vi "Memory.Pointer.Write Bytes.Safe.vi"(8 "error in (no error)":errorcluster, 9 "offset (0)":u64 format="%d bytes", 10 "buffer":u8[](array[numeric]) format="%02x", 11 "Pointer in":refnum<class "Memory.Pointer.Void.lvclass">) -> (0 "error out":errorcluster, 1 "offset dup":u64 format="%d bytes", 2 "buffer dup":u8[](array[numeric]) format="%02x", 3 "Pointer out":refnum<class "Memory.Pointer.Void.lvclass">)   [LabVIEW 2016, in "Memory Manager.lvlib" / "Memory.Pointer.Void.lvclass"]
uses:
  Memory.Pointer.Void.lvclass
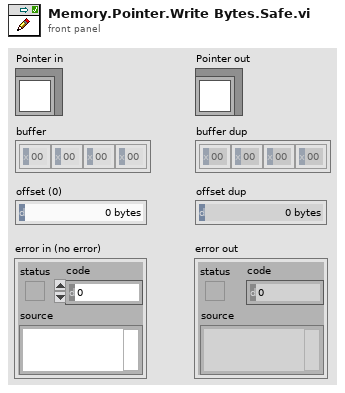
[diagram p1: front panel]
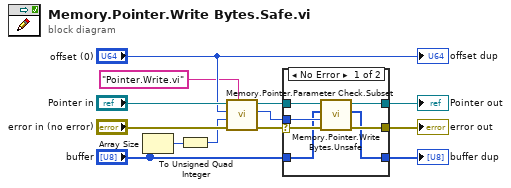
[diagram p0: block diagram]
diagram:
  n1 = Array Size(array="buffer") -> (size(s)=w11:i32)
  n2 = To Unsigned Quad Integer(1:w11) -> (0:w3:u64)
  n3 = call "Memory.Pointer.Parameter Check.Subset.vi"("calling vi name"="Pointer.Write.vi", "error in (no error)"="error in (no error)", "length"=w3, "offset"="offset (0)", "Pointer in"="Pointer in") -> ("error out"=w1:errorcluster, "offset out"=w4:u64, "Pointer out"=w5:refnum<class "Memory.Pointer.Void.lvclass">)  [unwired: 3 in, 1 out]
  n4 = case shown="No Error" w1 {
    selector: w1 -> [w15 w21]
    tunnel: [w19 w23] -> w13
    tunnel: [w18 w21] -> w12
    tunnel: [w17 w22] -> w10
    tunnel: "buffer" -> [w14 w22]
    tunnel: w5 -> [w20 w23]
    tunnel: w4 -> [w16 _]
    frame No Error {
      n5 = call "Memory.Pointer.Write Bytes.Unsafe.vi"("error in (no error)"=w15, "offset (0)"=w16, "buffer"=w14, "Pointer in"=w20) -> ("error out"=w18:errorcluster, "buffer dup"=w17:u8[], "Pointer out"=w19:refnum<class "Memory.Pointer.Void.lvclass">)  [unwired: 4 in, 1 out]
    }
    frame Error {
    }
  }
  "error out" <- w12
  "Pointer out" <- w13
  "buffer dup" <- w10
  "offset dup" <- "offset (0)"
